vi "GetPos.vi"(6 "Position 2":refnum<vi>, 8 "error in (no error)":errorcluster, 11 "Controlador in":refnum<class "Controlador.lvclass">) -> (0 "error out":errorcluster, 2 "Position":dbl, 3 "Controlador out":refnum<class "Controlador.lvclass">)   [LabVIEW 2011]
uses:
  Controlador.lvclass
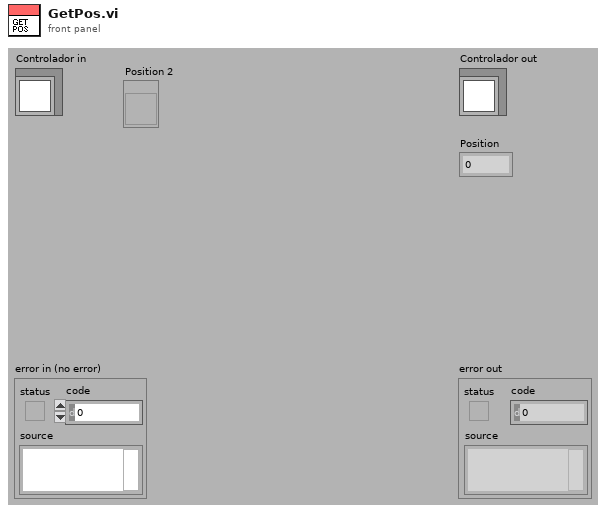
[diagram p1: front panel]
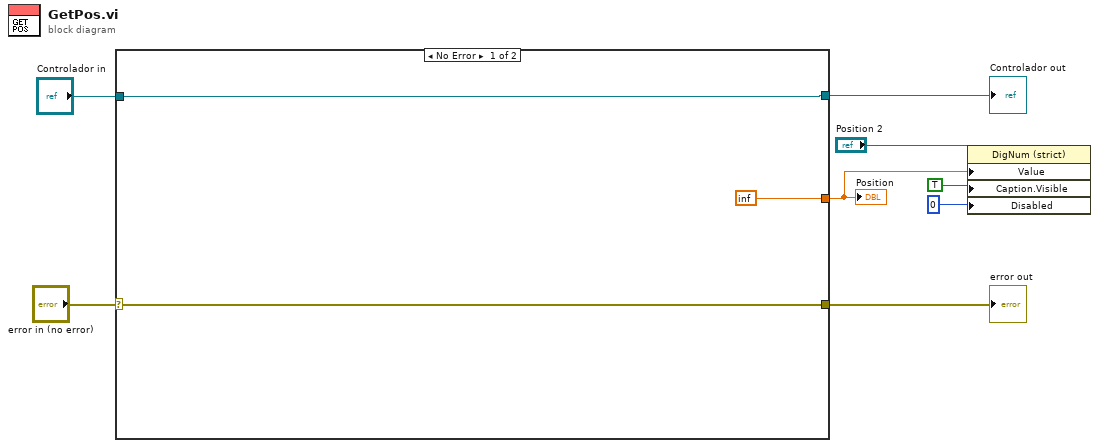
[diagram p0: block diagram]
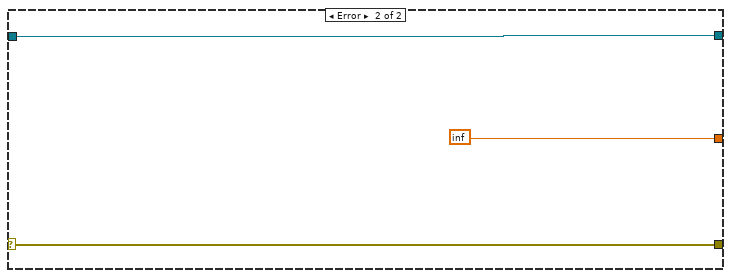
[diagram p2: hidden frame]
diagram:
  n1 = case shown="No Error" "error in (no error)" {
    selector: "error in (no error)" -> [w10 w13]
    tunnel: "Controlador in" -> [w11 w14]
    tunnel: [w10 w13] -> w6
    tunnel: [w11 w14] -> w7
    tunnel: [inf inf] -> w3
    frame No Error {
    }
    frame Error {
    }
  }
  "error out" <- w6
  "Controlador out" <- w7
  "Position" <- w3
  n2 = property class="DigNum (strict)"(reference="Position 2", "Value"=w3, "Caption.Visible"=TRUE, "Disabled"=u8 0) -> ()  [unwired: 1 in, 2 out]
